vi "Send Init.vi"(7 "Message Priority (Normal)":T2=enum."Normal", 8 "error in (no error)":errorcluster, 10 "Address":T1, 11 "Message Enqueuer":refnum<class "Message Enqueuer.lvclass">) -> (0 "error out":errorcluster, 3 "Message Enqueuer out":refnum<class "Message Enqueuer.lvclass">)   [LabVIEW 2023, in "ZWO_ASI.lvlib" / "Init Msg.lvclass"]
doc: "This VI sends the message to an actor."
uses:
  Init Msg.lvclass
  <vilib>/ActorFramework/Message Enqueuer/Message Enqueuer.lvclass
  <vilib>/ActorFramework/Message Enqueuer/Message Priority.ctl
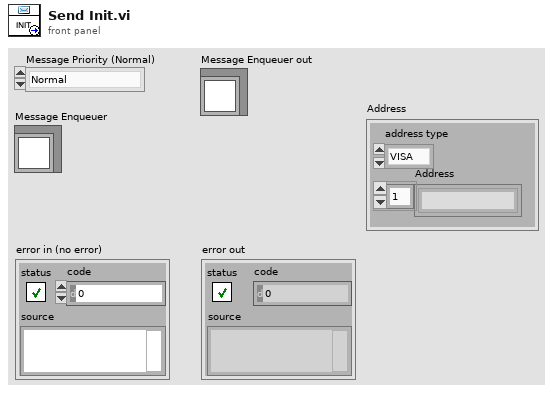
[diagram p1: front panel]
types:
  T1 = cluster{"address type":enum16{"VISA", "Index"}, "Address":string[]}
  T2 = typedef "Actor Framework.lvlib/Message Enqueuer.lvclass/Message Priority.ctl" = enum16{"Low", "Normal", "High"}
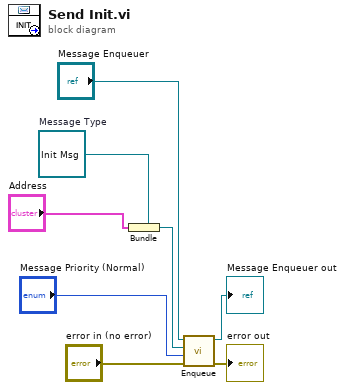
[diagram p0: block diagram]
diagram:
  w5 = refnum<class "Init Msg.lvclass"> refnum  # Message Type
  n1 = Bundle(cluster=w5, "Address") -> (w4:refnum<class "Init Msg.lvclass">)
  n2 = call <vilib>:"Enqueue.vi"("error in (no error)"="error in (no error)", "Message Priority (Normal)"="Message Priority (Normal)", "Message"=w4, "Message Enqueuer in"="Message Enqueuer") -> ("error out"=→"error out":errorcluster, "Message Enqueuer out"=→"Message Enqueuer out":refnum<class "Message Enqueuer.lvclass">)  [unwired: 6 in]
